vi "PopulateControlsFromCSV2 -Keep.vi"() -> ()   [LabVIEW 2019]
uses:
  <vilib>/Utility/file.llb/Read Delimited Spreadsheet (string).vi
panel:
  in  "Numeric1":dbl
  in  "Numeric2":dbl
  in  "Numeric3":dbl
  in  "Numeric4":dbl
  in  "Path":path=path "C:/Users/jbrus/Documents/GitHub/LabVIEW/3LabVIEWFeatures/PopulateControlsFromCSV/FileOutput.csv"
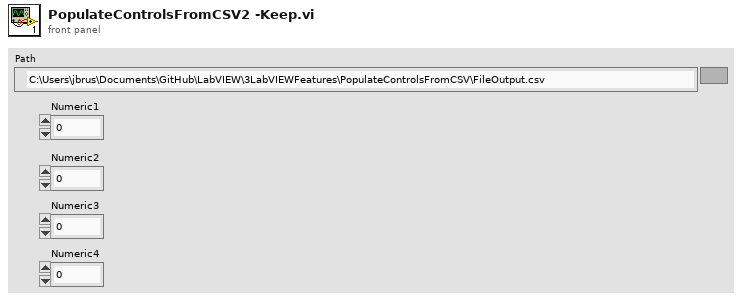
[diagram p1: front panel]
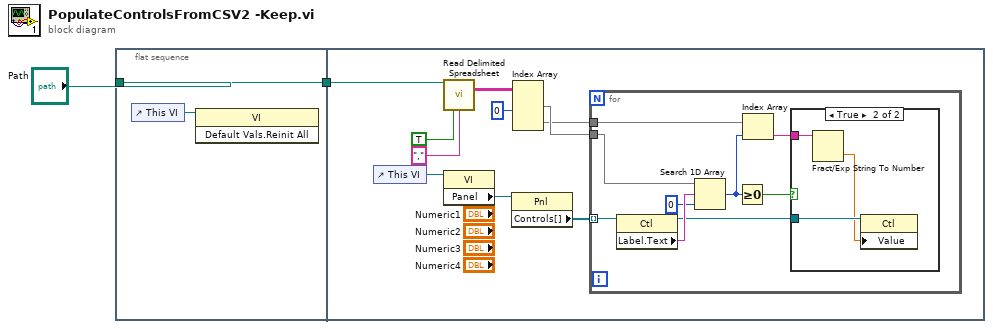
[diagram p0: block diagram]
diagram:
  n1 = flat-sequence {
    tunnel: [w3] -> w2
    tunnel: "Path" -> [w3]
    tunnel: w2 -> [w5]
    frame #0 {
      n2 = control-ref of="This VI"() -> (w4:refnum<vi>)
      n3 = invoke class="VI" method="Default Vals.Reinit All"(reference=w4) -> ()  [unwired: 2 in, 3 out]
    }
    frame #1 {
      n4 = control-ref of="This VI"() -> (w12:refnum<vi>)
      n5 = call-poly <vilib>:"Read Delimited Spreadsheet.vi"("file path (dialog if empty)"=w5, "transpose? (F)"=TRUE, "delimiter (\\t)"="," ("delimiter (\\t)")) -> ("all rows"=w9:string[][])  [unwired: 7 in, 5 out]
      n6 = property class="VI"(reference=w12) -> ("Panel"=w13:refnum<vi>)  [unwired: 1 in, 2 out]
      n7 = property class="Pnl"(reference=w13) -> ("Controls[]"=w14:refnum<vi>[])  [unwired: 1 in, 2 out]
      n8 = Index Array(array=w9, index (col) #1=0 ("disabled index (col)")) -> (element #1=w8:string[], element #2=w6:string[])  [unwired: 3 in]
      n9 = for {
        tunnel: w14 -> [w21] mode=indexing
        tunnel: w8 -> [w18]
        tunnel: w6 -> [w15]
        n10 = property class="Ctl"(reference=w21) -> (reference out=w20:refnum<vi>, "Label.Text"=w23:string)  [unwired: 1 in, 1 out]
        n11 = Search 1D Array(1D array=w18, element=w23, start index (0)=0) -> (index of element=w17:i32)
        n12 = Greater Or Equal To 0?(x=w17) -> (x >= 0?=w19:bool)
        n13 = Index Array(array=w15, index=w17) -> (element=w16:string)
        n14 = case shown="True" w19 {
          tunnel: w20 -> [_ w26]
          tunnel: w16 -> [_ w24]
          frame False {
          }
          frame True {
            n15 = Fract/Exp String To Number(string=w24) -> (number=w25:dbl)  [unwired: 3 in, 1 out]
            n16 = property class="Ctl"(reference=w26, "Value"=w25) -> ()  [unwired: 1 in, 2 out]
          }
        }
      }
    }
  }
